vi "DevicePublishOnDemandTagsRoutedMessage_Create.vi"(7 "Header":T1, 8 "error in (no error)":errorcluster, 10 "SendTo":string) -> (0 "error out":errorcluster, 3 "Message":T3)   [LabVIEW 2017]
uses:
  <vilib>/addons/InsightCM/MessageBus/Base/controls/Message.ctl
  <vilib>/addons/InsightCM/MessageBus/Base/controls/MessageHeader.ctl
  <vilib>/addons/InsightCM/MessageBus/Base/controls/KeyValuePair.ctl
  <vilib>/addons/InsightCM/MessageBus/Base/controls/MessageClassType.ctl
  <vilib>/addons/InsightCM/Utilities/PropertyHelpers/PropertyHelpers.lvlib
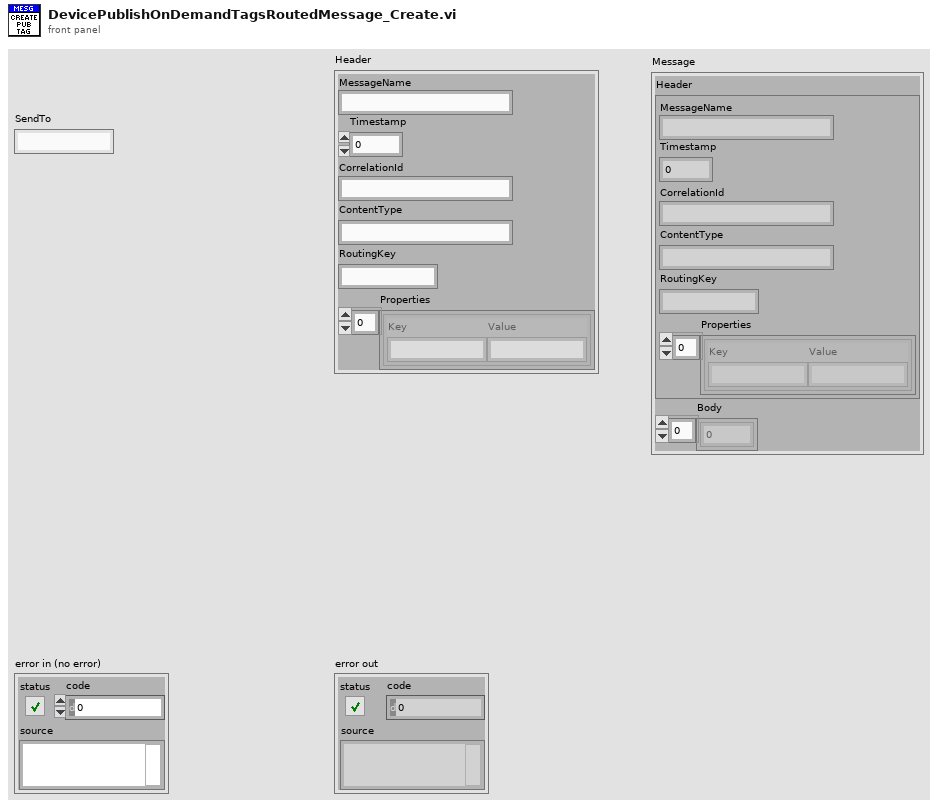
[diagram p1: front panel]
types:
  T1 = typedef "MessageHeader.ctl" = cluster{"MessageName":string, "Timestamp":i64, "CorrelationId":string, "ContentType":string, "RoutingKey":string, "Properties":T2[]}
  T2 = typedef "KeyValuePair.ctl" = cluster{"Key":string, "Value":string}
  T3 = typedef "Message.ctl" = cluster{"Header":T1, "Body":u8[]}
  T4 = typedef "MessageClassType.ctl" = enum16{"Request", "Response", "Broadcast", "RoutedMessage"}
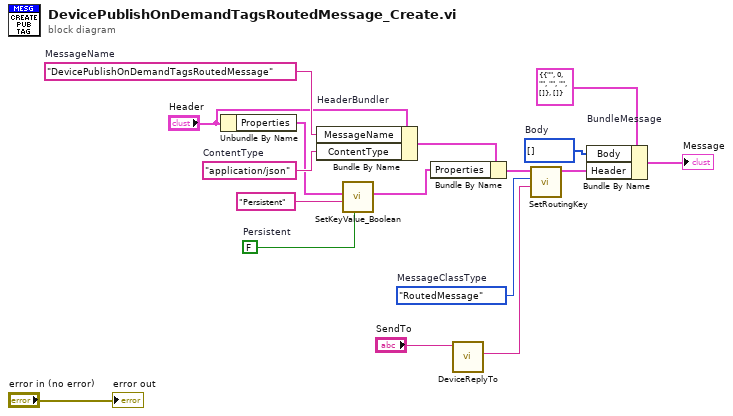
[diagram p0: block diagram]
diagram:
  w16 = u8[] []  # Body
  w14 = MessageClassType."RoutedMessage"  # MessageClassType
  w9 = FALSE  # Persistent
  w15 = "DevicePublishOnDemandTagsRoutedMessage"  # MessageName
  w12 = "application/json"  # ContentType
  n1 = Unbundle By Name("Header") -> ("Properties"=w11:T2[])
  n2 = Bundle By Name "HeaderBundler"(cluster="Header", "MessageName"=w15, "ContentType"=w12) -> (w6:T1)
  n3 = call <vilib>:"SetKeyValue_Boolean.vi"("value"=w9, "key"="Persistent" ("Key"), "key value pairs"=w11) -> ("key value pairs out"=w5:T2[])  [unwired: 8 in]
  n4 = Bundle By Name(cluster=w6, "Properties"=w5) -> (w7:T1)
  n5 = call <vilib>:"DeviceReplyTo.vi"("Device"="SendTo") -> ("ReplyTo"=w1:string)  [unwired: 10 in]
  n6 = call <vilib>:"SetRoutingKey.vi"("SendTo"=w1, "MessageClassType"=w14, "Message Header in"=w7) -> ("Message Header out"=w8:T1)  [unwired: 8 in]
  n7 = Bundle By Name "BundleMessage"(cluster=T3 {"Header"={"MessageName"="", "Timestamp"=0, "CorrelationId"="", "ContentType"="", "RoutingKey"="", "Properties"=[]}, "Body"=[]} ("Message"), "Body"=w16, "Header"=w8) -> (→"Message":T3)
  "error out" <- "error in (no error)"
